vi "writeToXML.vi"(8 "error in (no error)":errorcluster, 10 "ClassLabel":string, 11 "ADCWavelength in":refnum<class "ADCWavelength.lvclass">) -> (0 "error out":errorcluster, 2 "XML out":string, 3 "ADCWavelength out":refnum<class "ADCWavelength.lvclass">)   [LabVIEW 2014, in "TCSDataDefinitions.lvlib" / "TCSAtmosphericDispersionCommand.lvlib" / "ADCWavelength.lvclass"]
uses:
  ADCWavelength.lvclass
  <userlib>/Common/UnitsAndXML/FlattenItemWithUnitToXML/FlattenLengthToXML/LengthUnit.ctl
  ADCWavelength.lvclass/ADCWavelength.ctl
  TCSAtmosphericDispersionCommand/TCSAtmosphericDispersionCommand.lvclass
  <userlib>/Common/UnitsAndXML/UnitsAndXML.lvlib
  <userlib>/Common/XML/XMLGenerator/XMLGenerator.lvclass
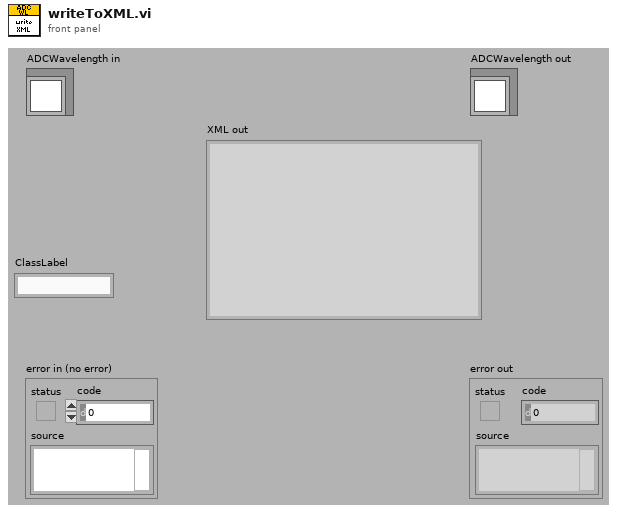
[diagram p1: front panel]
types:
  T1 = typedef "UnitsAndXML.lvlib/LengthUnit.ctl" = enum16{"m", "Angstrom", "AU", "chain", "cm", "cubit", "fathom", "fermi", "ft", "furlong", "hubble", "in", "ly", "mi", "mm", "rod", "um", "yd"}
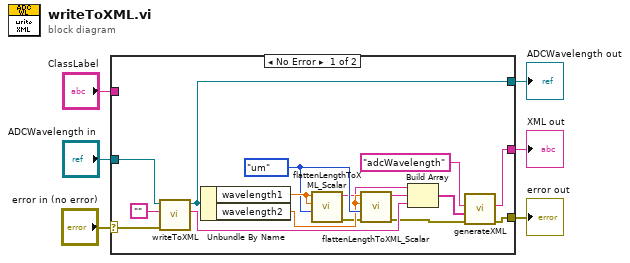
[diagram p0: block diagram]
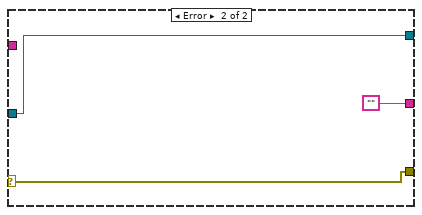
[diagram p2: hidden frame]
diagram:
  n1 = case shown="No Error" "error in (no error)" {
    selector: "error in (no error)" -> [w9 w25]
    tunnel: [w10 w25] -> w5
    tunnel: [w17 w24] -> w3
    tunnel: "ADCWavelength in" -> [w18 w24]
    tunnel: "ClassLabel" -> [_ _]
    tunnel: [w7 ""] -> w1
    frame No Error {
      w21 = LengthUnit."um" ("lengthUnitInXML")
      n2 = call-parent "writeToXML.vi"("error in (no error)"=w9, "ClassLabel"="", "TCSAtmosphericDispersionCommand in"=w18) -> ("XML out"=w16:string, "TCSAtmosphericDispersionCommand out"=w17:refnum<class "ADCWavelength.lvclass">)  [unwired: 6 in, 1 out]
      n3 = Unbundle By Name(w17) -> ("wavelength1"=w22:dbl[unit], "wavelength2"=w20:dbl[unit])
      n4 = call <userlib>:"flattenLengthToXML_Scalar.vi"("lengthUnitInXML"=w21, "lengthAgain"=w22, "length"=w22) -> ("error out"=w19:errorcluster, "xmlString"=w14:string)  [unwired: 7 in]
      n5 = call <userlib>:"flattenLengthToXML_Scalar.vi"("error in (no error)"=w19, "lengthUnitInXML"=w21, "lengthAgain"=w20, "length"=w20) -> ("error out"=w11:errorcluster, "xmlString"=w15:string)  [unwired: 6 in]
      n6 = Build Array(w14, w15, w16) -> (w13:string[])
      n7 = call <userlib>:"generateXML.vi"("error in"=w11, "childrenXML"=w13, "elementName"="adcWavelength" ("Class Label")) -> ("error out"=w10:errorcluster, "XML out"=w7:string)  [unwired: 6 in, 1 out]
    }
    frame Error {
    }
  }
  "error out" <- w5
  "ADCWavelength out" <- w3
  "XML out" <- w1
